vi "Set Termination TTL.vi"(8 "error in (no error)":errorcluster, 9 "TTL":refnum<class "TTLController.lvclass">[](array[class]), 10 "termIndex":i32, 11 "State in":refnum<class "State.lvclass">) -> (0 "error out":errorcluster, 3 "State out":refnum<class "State.lvclass">)   [LabVIEW 2015, in "State.lvclass"]
uses:
  State.lvclass
  TTL VIs/Control Classes/Base Class/TTLController.lvclass
  State.lvclass/State.ctl
  Termination/Termination.lvclass/Termination.ctl
  Termination/Write TTL.vi
  Termination/Termination.lvclass
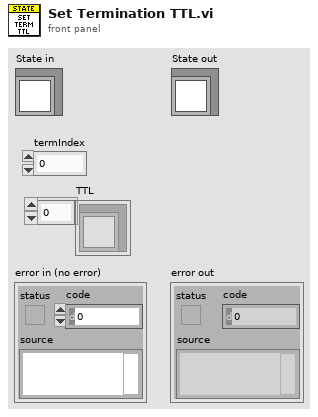
[diagram p1: front panel]
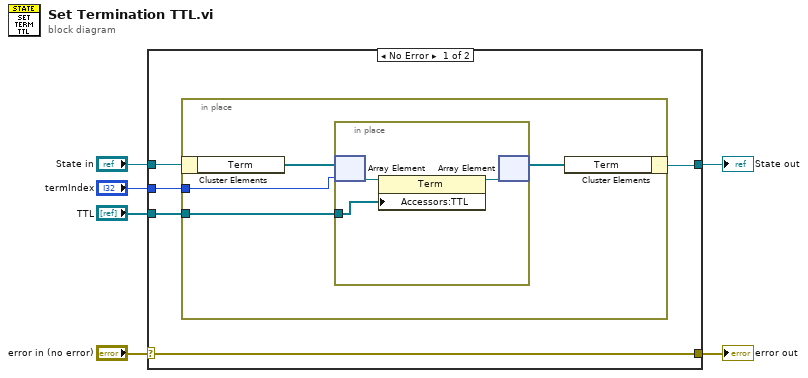
[diagram p0: block diagram]
diagram:
  n1 = case shown="No Error" "error in (no error)" {
    selector: "error in (no error)" -> [w11 w20]
    tunnel: [w11 w20] -> w5
    tunnel: [w8 w19] -> w3
    tunnel: "State in" -> [w10 w19]
    tunnel: "termIndex" -> [w9 _]
    tunnel: "TTL" -> [w7 _]
    frame No Error {
      n2 = in-place {
        in-place-border: w9 -> [w14]
        in-place-border: w7 -> [w12]
        n3 = in-place-cluster #1(w10) -> ("Term"=w15:refnum<class "Termination.lvclass">[])
        n4 = in-place {
          in-place-border: w12 -> [w16]
          n5 = in-place-array #2(w15, w14) -> (w18:refnum<class "Termination.lvclass">)
          n6 = property class="Term"(reference=w18, "Accessors:TTL"=w16) -> (reference out=w17:refnum<class "Termination.lvclass">)  [unwired: 1 in, 1 out]
          n7 = in-place-array #2(w17) -> (w13:refnum<class "Termination.lvclass">[])  [unwired: 1 out]
        }
        n8 = in-place-cluster #1("Term"=w13) -> (w8:refnum<class "State.lvclass">)
      }
    }
    frame Error {
    }
  }
  "error out" <- w5
  "State out" <- w3
